vi "pwm_to_angle_conversion.vi"(6 "theta high":dbl, 7 "theta low":dbl, 9 "pwm low":dbl, 10 "pwm":dbl, 11 "pwm high":dbl) -> (3 "Angle":dbl)   [LabVIEW 2017]
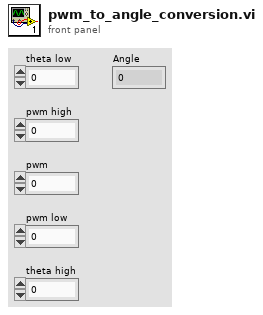
[diagram p1: front panel]
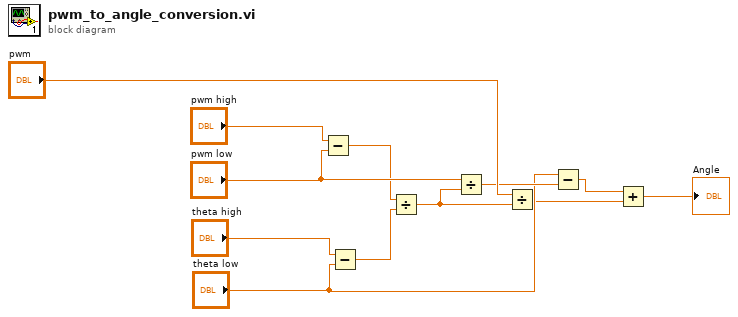
[diagram p0: block diagram]
diagram:
  n1 = Subtract(x="pwm high", y="pwm low") -> (x-y=w3:dbl)
  n2 = Subtract(x="theta high", y="theta low") -> (x-y=w4:dbl)
  n3 = Divide(x=w3, y=w4) -> (x/y=w6:dbl)
  n4 = Divide(x="pwm low", y=w6) -> (x/y=w9:dbl)
  n5 = Divide(x="pwm", y=w6) -> (x/y=w5:dbl)
  n6 = Subtract(x="theta low", y=w9) -> (x-y=w10:dbl)
  n7 = Add(x=w10, y=w5) -> (x+y=→"Angle":dbl)
